vi "Init.vi"(0 "Session":T3="cam0", 5 "error in":errorcluster) -> (6 "Device Serial Number":string, 7 "Exposure Time - READ":dbl, 8 "Message":string, 10 "Gain Min":i64, 12 "Gain Max":i64, 13 "Gain - READ":i64, 14 "IMAQdx Session OUT":T3, 15 "Success?":bool, 18 "error out":errorcluster, 19 "error out  - closing camera":errorcluster)   [LabVIEW 2014]
uses:
  <vilib>/userdefined/High Color/IMAQdx.ctl
  <vilib>/vision/driver/IMAQdx.llb/IMAQdx Attribute Type.ctl
  <vilib>/vision/driver/IMAQdx.llb/IMAQdx Camera Control Mode.ctl
  <vilib>/vision/driver/IMAQdx.llb/IMAQdx Acquisition Mode.ctl
  <vilib>/vision/driver/NI_Vision_Acquisition_Software.lvlib
  <resource>/objmgr/imaqdx.rc
panel:
  out "IncI64":i64
  out "IncDBL":dbl
  out "Units":string
  in  "ValueU32":u32=2
  out "EnumValues[]":u32[](array[numeric])
  out "EnumStrings[]":string[](array[string])
  out "New exposure":dbl
  out "error out 2":errorcluster
  out "Attribute Information Array":T2(array[cluster])
  out "ModelName":string
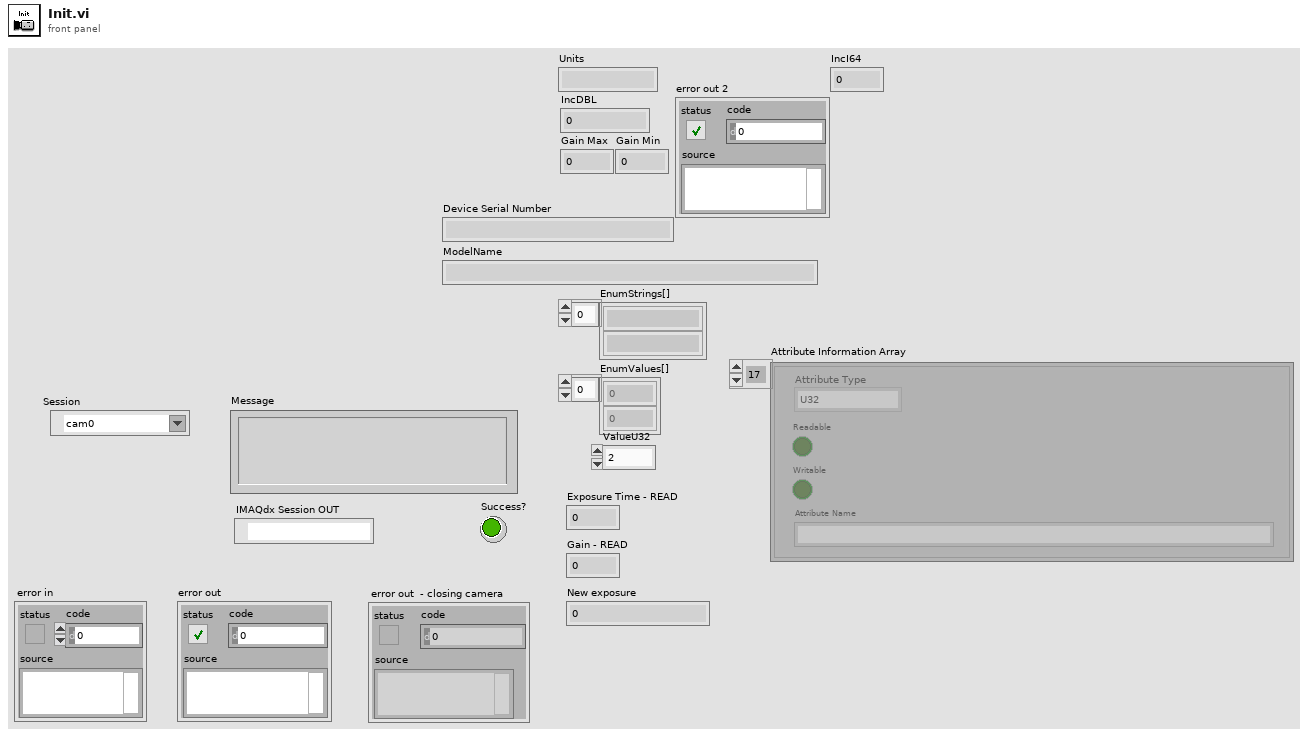
[diagram p1: front panel]
types:
  T1 = typedef "NI_Vision_Acquisition_Software.lvlib/IMAQdx Attribute Type.ctl" = enum32{"U32", "I64", "DBL", "String", "Enum", "Bool", "Command"}
  T2 = cluster{"Attribute Type":T1, "Readable":bool, "Writable":bool, "Attribute Name":string}[]
  T3 = typedef "IMAQdx.ctl" = refnum<k21>
  T4 = typedef "NI_Vision_Acquisition_Software.lvlib/IMAQdx Camera Control Mode.ctl" = enum32{"Controller", "Listener"}
  T5 = typedef "NI_Vision_Acquisition_Software.lvlib/IMAQdx Acquisition Mode.ctl" = enum32{"One Shot", "Continuous"}
  T6 = cluster{"Type":u32, "Version":u32, "Flags":u32, "SerialNumberHigh":u32, "SerialNumberLow":u32, "BusType":u32, "InterfaceName":string, "VendorName":string, "ModelName":string, "CameraFileName":string, "CameraAttributeURL":string}[]
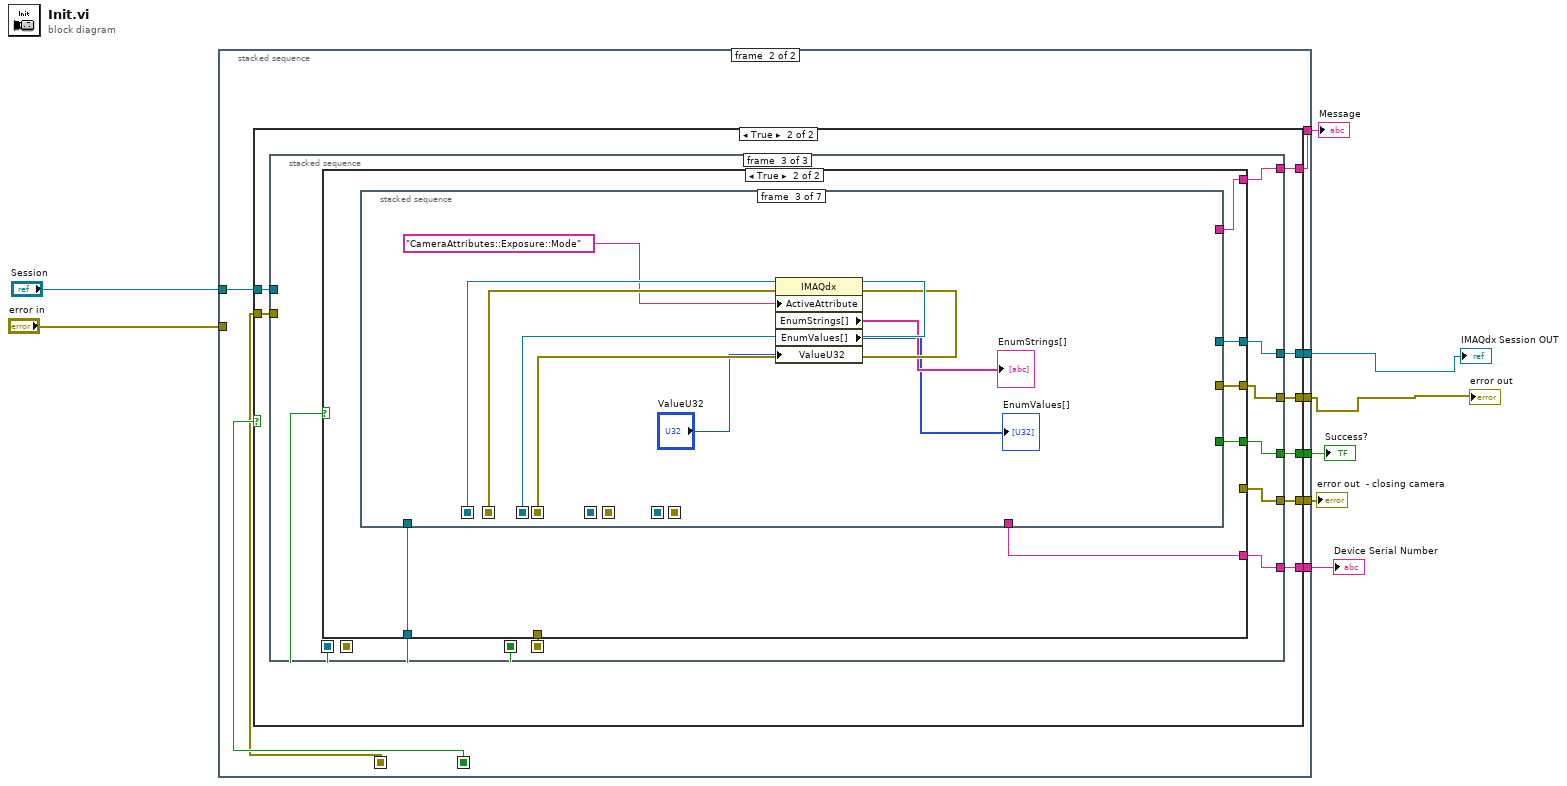
[diagram p0: block diagram]
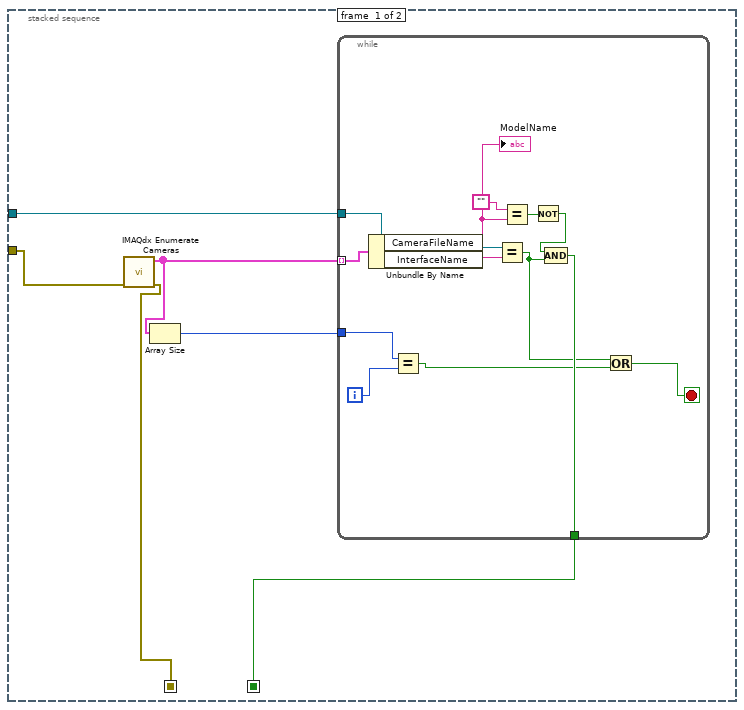
[diagram p2: hidden frame]
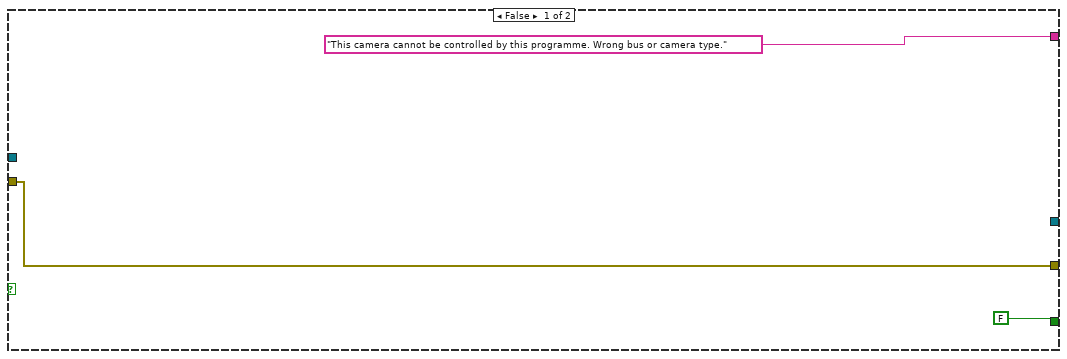
[diagram p3: hidden frame]
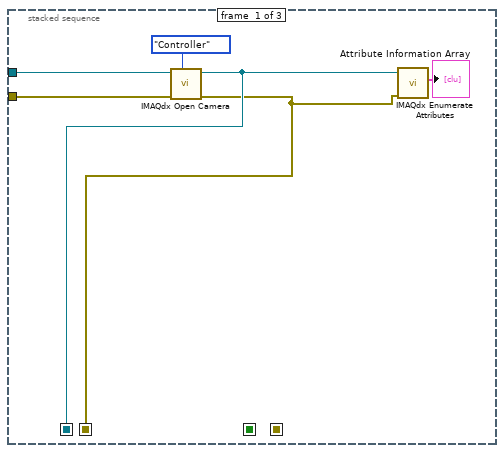
[diagram p4: hidden frame]
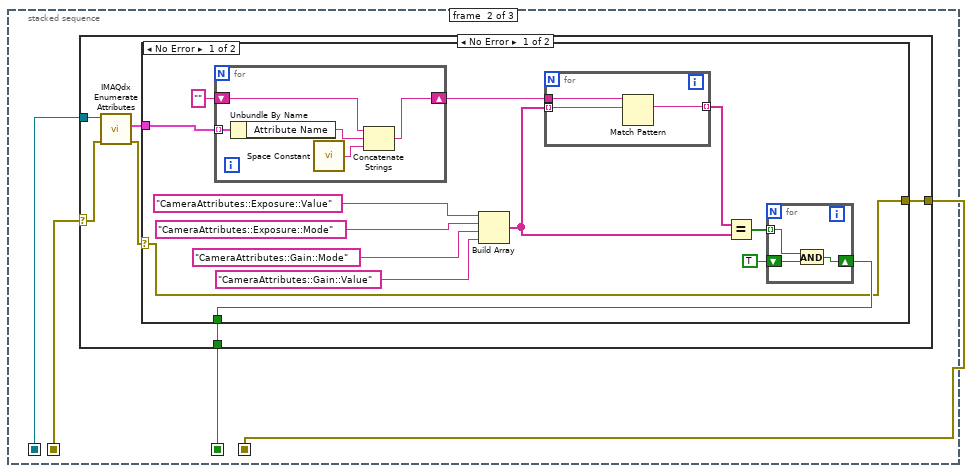
[diagram p5: hidden frame]
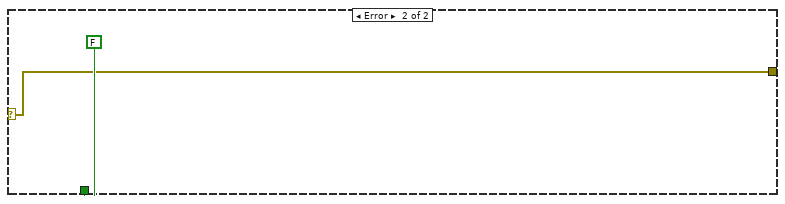
[diagram p6: hidden frame]
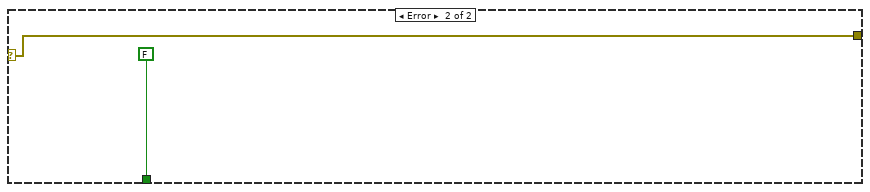
[diagram p7: hidden frame]
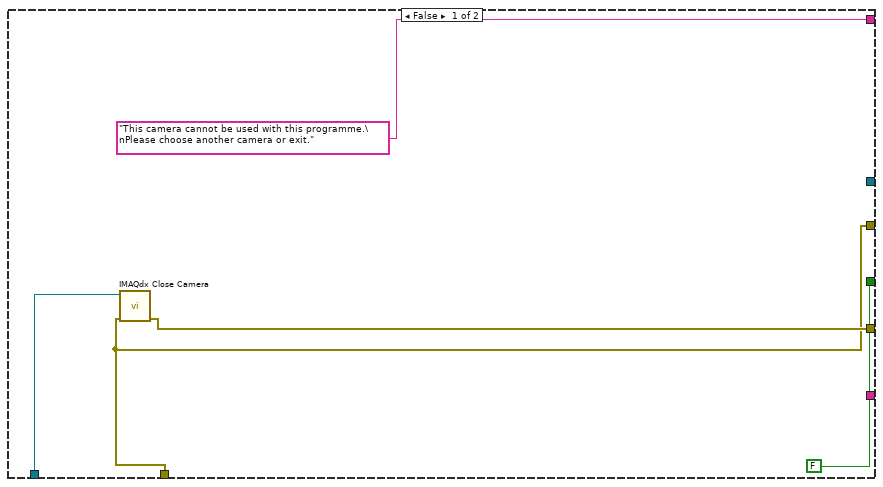
[diagram p8: hidden frame]
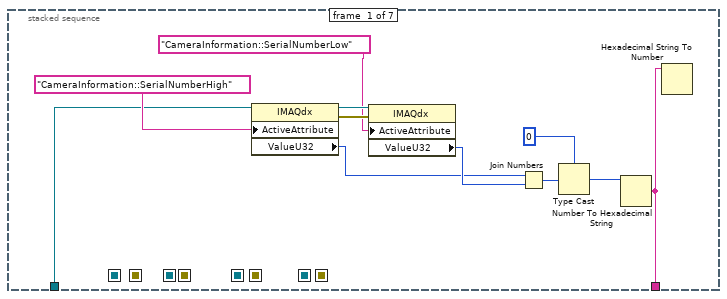
[diagram p9: hidden frame]
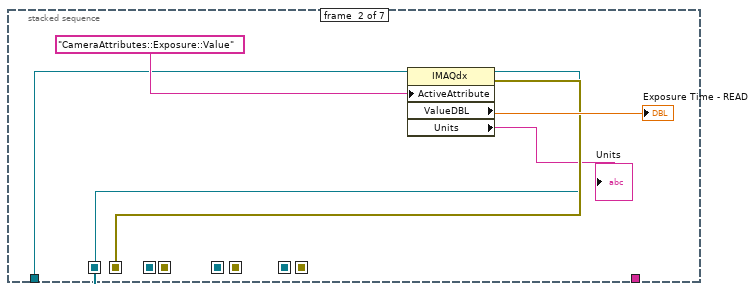
[diagram p10: hidden frame]
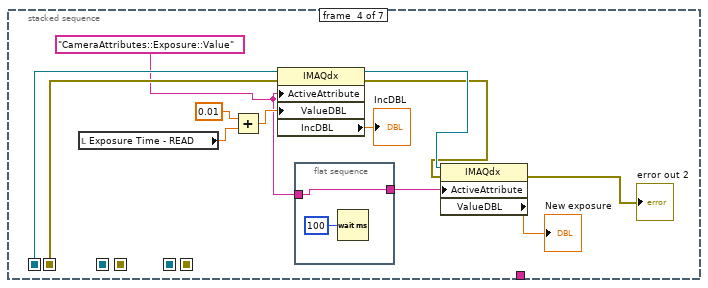
[diagram p11: hidden frame]
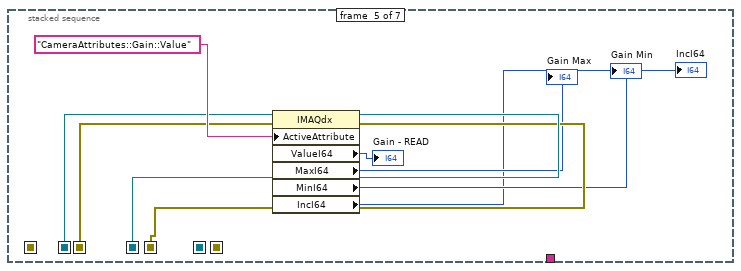
[diagram p12: hidden frame]
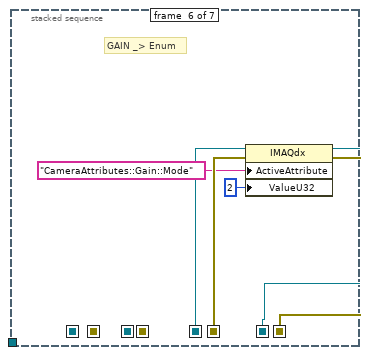
[diagram p13: hidden frame]
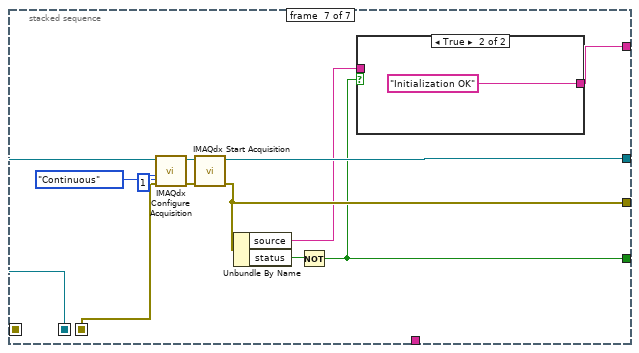
[diagram p14: hidden frame]
diagram:
  n1 = stacked-sequence {
    seq-local: [w13 _] -> [_ w31]
    seq-local: [w9 _] -> [_ w28]
    tunnel: [_ w36] -> w8
    tunnel: [_ w35] -> w2
    tunnel: [_ w30] -> w1
    tunnel: [_ w34] -> w7
    tunnel: "Session" -> [w14 w33]
    tunnel: [_ w32] -> w5
    tunnel: "error in" -> [w10 _]
    tunnel: [_ w29] -> w3
    frame #0 {
      n2 = call <vilib>:"IMAQdx Enumerate Cameras.vi"("error in"=w10) -> ("error out"=w9:errorcluster, "Camera Information Array"=w12:T6)  [unwired: 9 in]
      n3 = Array Size(array=w12) -> (size(s)=w11:i32)
      n4 = while {
        tunnel: w12 -> [w27] mode=indexing
        tunnel: w14 -> [w26]
        tunnel: [w22] -> w13
        tunnel: w11 -> [w23]
        i -> [w24]
        stop <- w20 stop-if-true
        n5 = Unbundle By Name(w27) -> ("CameraFileName"=w19:string, "InterfaceName"=w25:string)
        "ModelName" <- w19
        n6 = Equal?(x=w23, y=w24) -> (x = y?=w21:bool)
        n7 = Equal?(x=w26, y=w25) -> (x = y?=w15:bool)
        n8 = Equal?(x="", y=w19) -> (x = y?=w17:bool)
        n9 = Not(x=w17) -> (.not. x?=w16:bool)
        n10 = Compound Arithmetic op=AND(w16, w15) -> (w22:bool)
        n11 = Or(x=w15, y=w21) -> (x .or. y?=w20:bool)
      }
    }
    frame #1 {
      n12 = case shown="True" w31 {
        tunnel: ["This camera cannot be controlled by this programme. Wrong bus or camera type." ("source") w47] -> w36
        tunnel: [_ w46] -> w35
        tunnel: [FALSE w45] -> w34
        tunnel: w33 -> [_ w44]
        tunnel: [_ w43] -> w32
        tunnel: w28 -> [w38 w42]
        tunnel: [w38 w40] -> w30
        tunnel: [_ w41] -> w29
        frame False {
        }
        frame True {
          n13 = stacked-sequence {
            seq-local: [w49 _ _] -> [_ w55 _]
            seq-local: [w50 _ _] -> [_ w57 w100]
            seq-local: [_ w56 _] -> [_ _ w99]
            seq-local: [_ w54 _] -> [_ _ w93]
            tunnel: [_ _ w98] -> w47
            tunnel: [_ _ w97] -> w46
            tunnel: [_ _ w96] -> w45
            tunnel: w44 -> [w52 _ _]
            tunnel: [_ _ w95] -> w43
            tunnel: w42 -> [w51 _ _]
            tunnel: [_ _ w94] -> w41
            tunnel: [_ _ w92] -> w40
            frame #0 {
              n14 = call <vilib>:"IMAQdx Open Camera.vi"("Camera Control Mode"=IMAQdx_Camera_Control_Mode."Controller", "error in"=w51, "Session In"=w52) -> ("error out"=w49:errorcluster, "Session Out"=w50:T3)  [unwired: 7 in]
              n15 = call <vilib>:"IMAQdx Enumerate Attributes.vi"("error in"=w49, "Session In"=w50) -> ("Attribute Information Array"=→"Attribute Information Array":T2)  [unwired: 7 in, 2 out]
            }
            frame #1 {
              n16 = case shown="No Error" w55 {
                selector: w55 -> [w59 w90]
                tunnel: w57 -> [w63 _]
                tunnel: [w61 FALSE] -> w56
                tunnel: [w58 w90] -> w54
                frame No Error {
                  n17 = call <vilib>:"IMAQdx Enumerate Attributes.vi"("error in"=w59, "Session In"=w63) -> ("error out"=w60:errorcluster, "Attribute Information Array"=w62:T2)  [unwired: 7 in, 1 out]
                  n18 = case shown="No Error" w60 {
                    selector: w60 -> [w64 w88]
                    tunnel: w62 -> [w76 _]
                    tunnel: [w66 FALSE] -> w61
                    tunnel: [w64 w88] -> w58
                    frame No Error {
                      n19 = for {
                        tunnel: w76 -> [w87] mode=indexing
                        shift-right: [w84] -> w70
                        shift-left: "" -> [w83]
                        n20 = Unbundle By Name(w87) -> ("Attribute Name"=w86:string)
                        n21 = call <vilib>:"Space Constant.vi"() -> ("String"=w85:string)
                        n22 = Concatenate Strings(w83, w86, w85) -> (w84:string)
                      }
                      n23 = Build Array("CameraAttributes::Exposure::Value" ("Attribute Name"), "CameraAttributes::Exposure::Mode" ("Attribute Name"), "CameraAttributes::Gain::Mode" ("Attribute Name"), "CameraAttributes::Gain::Value" ("Attribute Name")) -> (w65:string[])
                      n24 = for {
                        tunnel: w70 -> [w82]
                        tunnel: w65 -> [w81] mode=indexing
                        tunnel: [w80] -> w69 mode=indexing
                        n25 = Match Pattern(string=w82, regular expression=w81) -> (match substring=w80:string)  [unwired: 1 in, 3 out]
                      }
                      n26 = Equal?(x=w69, y=w65) -> (x = y?=w68:bool[])
                      n27 = for {
                        tunnel: w68 -> [w79] mode=indexing
                        shift-right: [w77] -> w66
                        shift-left: TRUE -> [w78]
                        n28 = And(x=w79, y=w78) -> (x .and. y?=w77:bool)
                      }
                    }
                    frame Error {
                    }
                  }
                }
                frame Error {
                }
              }
            }
            frame #2 {
              n29 = case shown="True" w99 {
                tunnel: w100 -> [w101 w111]
                tunnel: ["This camera cannot be used with this programme.\nPlease choose another camera or exit." w107] -> w98
                tunnel: [_ w110] -> w97
                tunnel: [w102 w109] -> w92
                tunnel: [FALSE w108] -> w96
                tunnel: [w103 _] -> w95
                tunnel: [_ w106] -> w94
                tunnel: w93 -> [w102 _]
                frame False {
                  n30 = call <vilib>:"IMAQdx Close Camera.vi"("error in"=w102, "Session In"=w101) -> ("error out"=w103:errorcluster)  [unwired: 9 in]
                }
                frame True {
                  n31 = stacked-sequence {
                    seq-local: [_ w125 _ _ _ _ _] -> [_ _ w135 _ _ _ _]
                    seq-local: [_ w124 _ _ _ _ _] -> [_ _ w136 _ _ _ _]
                    seq-local: [_ _ w134 _ _ _ _] -> [_ _ _ w148 w157 _ _]
                    seq-local: [_ _ w133 _ _ _ _] -> [_ _ _ w147 w156 _ _]
                    seq-local: [_ _ _ _ w155 _ _] -> [_ _ _ _ _ w165 _]
                    seq-local: [_ _ _ _ w154 _ _] -> [_ _ _ _ _ w164 _]
                    seq-local: [_ _ _ _ _ w163 _] -> [_ _ _ _ _ _ w170]
                    seq-local: [_ _ _ _ _ w162 _] -> [_ _ _ _ _ _ w169]
                    tunnel: w111 -> [w121 w127 _ _ _ _ _]
                    tunnel: [_ _ _ _ _ _ w173] -> w110
                    tunnel: [_ _ _ _ _ _ w172] -> w109
                    tunnel: [_ _ _ _ _ _ w168] -> w108
                    tunnel: [_ _ _ _ _ _ w167] -> w107
                    tunnel: [w112 _ _ _ _ _ _] -> w106
                    frame #0 {
                      n32 = property class="IMAQdx"(reference=w121, "ActiveAttribute"="CameraInformation::SerialNumberHigh" ("Attribute Name")) -> (reference out=w120:T3, error out=w119:errorcluster, "ValueU32"=w114:u32)  [unwired: 1 in]
                      n33 = property class="IMAQdx"(reference=w120, error in=w119, "ActiveAttribute"="CameraInformation::SerialNumberLow" ("Attribute Name")) -> ("ValueU32"=w117:u32)  [unwired: 2 out]
                      n34 = Join Numbers(hi=w114, lo=w117) -> ((hi.lo)=w116:u64)
                      n35 = Type Cast(type=u64 0 ("(hi.lo)"), x=w116) -> (*(type *) &x=w113:u64)
                      n36 = Number To Hexadecimal String(2:w113) -> (0:w112:string)  [unwired: 1 in]
                      n37 = Hexadecimal String To Number(string=w112) -> ()  [unwired: 2 in, 2 out]
                    }
                    frame #1 {
                      n38 = property class="IMAQdx"(reference=w127, "ActiveAttribute"="CameraAttributes::Exposure::Value" ("Attribute Name")) -> (reference out=w124:T3, error out=w125:errorcluster, "ValueDBL"=→"Exposure Time - READ":dbl, "Units"=→"Units":string)  [unwired: 1 in]
                    }
                    frame #2 {
                      n39 = property class="IMAQdx"(reference=w136, error in=w135, "ActiveAttribute"="CameraAttributes::Exposure::Mode" ("Attribute Name"), "ValueU32"="ValueU32") -> (reference out=w134:T3, error out=w133:errorcluster, "EnumStrings[]"=→"EnumStrings[]":string[], "EnumValues[]"=→"EnumValues[]":u32[])
                    }
                    frame #3 {
                      w139 = "CameraAttributes::Exposure::Value" ("Attribute Name")
                      n40 = local read "Exposure Time - READ"() -> (w145:dbl)
                      n41 = Add(x=0.01 ("Exposure Time - READ"), y=w145) -> (x+y=w144:dbl)
                      n42 = property class="IMAQdx"(reference=w148, error in=w147, "ActiveAttribute"=w139, "ValueDBL"=w144) -> (reference out=w143:T3, error out=w142:errorcluster, "IncDBL"=→"IncDBL":dbl)
                      n43 = flat-sequence {
                        tunnel: w139 -> [w150]
                        tunnel: [w150] -> w138
                        frame #0 {
                          n44 = Wait (ms)(milliseconds to wait=u32 100) -> ()  [unwired: 1 out]
                        }
                      }
                      n45 = property class="IMAQdx"(reference=w143, error in=w142, "ActiveAttribute"=w138) -> (error out=→"error out 2":errorcluster, "ValueDBL"=→"New exposure":dbl)  [unwired: 1 out]
                    }
                    frame #4 {
                      n46 = property class="IMAQdx"(reference=w157, error in=w156, "ActiveAttribute"="CameraAttributes::Gain::Value") -> (reference out=w155:T3, error out=w154:errorcluster, "ValueI64"=→"Gain - READ":i64, "MaxI64"=→"Gain Max":i64, "MinI64"=→"Gain Min":i64, "IncI64"=→"IncI64":i64)
                    }
                    frame #5 {
                      # "GAIN _> Enum"
                      n47 = property class="IMAQdx"(reference=w165, error in=w164, "ActiveAttribute"="CameraAttributes::Gain::Mode" ("Attribute Name"), "ValueU32"=u32 2) -> (reference out=w163:T3, error out=w162:errorcluster)
                    }
                    frame #6 {
                      n48 = call <vilib>:"IMAQdx Configure Acquisition.vi"("error in"=w169, "Number of Buffers"=1, "Continuous?"=IMAQdx_Acquisition_Mode."Continuous", "Session In"=w170) -> ("error out"=w176:errorcluster, "Session Out"=w175:T3)  [unwired: 6 in]
                      n49 = call <vilib>:"IMAQdx Start Acquisition.vi"("error in"=w176, "Session In"=w175) -> ("error out"=w172:errorcluster, "Session Out"=w173:T3)  [unwired: 8 in]
                      n50 = Unbundle By Name(w172) -> ("source"=w166:string, "status"=w171:bool)
                      n51 = Not(x=w171) -> (.not. x?=w168:bool)
                      n52 = case shown="True" w168 {
                        tunnel: [w178 "Initialization OK"] -> w167
                        tunnel: w166 -> [w178 _]
                        frame False {
                        }
                        frame True {
                        }
                      }
                    }
                  }
                }
              }
            }
          }
        }
      }
    }
  }
  "Message" <- w8
  "Success?" <- w7
  "error out  - closing camera" <- w5
  "Device Serial Number" <- w3
  "error out" <- w1
  "IMAQdx Session OUT" <- w2
